vi "Auton_S3_Left_Scale.vi"   [LabVIEW 2017]
uses:
  <vilib>/Rock Robotics/WPI/Utilities/WPI_GetSetVariantRefNum.vi
  Robot Global Data.vi
  <vilib>/Rock Robotics/WPI/RobotDrive/WPI_RobotDriveArcadeDrive_Standard(NoSaturation).vi
types:
  T1 = typedef "WPI_RobotDriveDevRef.ctl" = cluster{"DevStatus":errorcluster, "Motors[]":T2[], "Square Inputs":bool, "Max Output":dbl}
  T2 = typedef "WPI_MotorControlDeviceRef.ctl" = cluster{"DeviceStatus":errorcluster, "Type":T3, "PWM":cluster{"PWM Channel":T4, "DeadBand":T5}, "CAN":cluster{"Device Number":u8, "SetOutput VI Ref":variant, "GetOutput VI Ref":variant, "Enable VI Ref":variant, "Disable VI Ref":variant, "Data":variant}, "Invert":bool, "DIO PWM":cluster{"PWM \"Enable\" Channel":T4, "DIOChannel":T6, "PWM Rate":dbl}}
  T3 = typedef "WPI_MotorControlType.ctl" = enum16{"PWM", "CAN", "DIO PWM"}
  T4 = typedef "FPGA_DIOPWMChannel.ctl" = enum8{"PWM 0", "PWM 1", "PWM 2", "PWM 3", "PWM 4", "PWM 5", "PWM 6", "PWM 7", "PWM 8", "PWM 9", "PWM MXP 0", "PWM MXP 1", "PWM MXP 2", "PWM MXP 3", "PWM MXP 4", "PWM MXP 5", "PWM MXP 6", "PWM MXP 7", "PWM MXP 8", "PWM MXP 9", "Invalid"}
  T5 = typedef "WPI_PWMDeadband.ctl" = cluster{"Name":string, "maxPositivePwm":i32, "minPositivePwm":i32, "centerPwm":i32, "maxNegativePwm":i32, "minNegativePwm":i32, "angularRange":u16}
  T6 = typedef "FPGA_DIOChannel.ctl" = enum8{"DIO 0", "DIO 1", "DIO 2", "DIO 3", "DIO 4", "DIO 5", "DIO 6", "DIO 7", "DIO 8", "DIO 9", "DIO MXP 0", "DIO MXP 1", "DIO MXP 2", "DIO MXP 3", "DIO MXP 4", "DIO MXP 5", "DIO MXP 6", "DIO MXP 7", "DIO MXP 8", "DIO MXP 9", "DIO MXP 10", "DIO MXP 11", "DIO MXP 12", "DIO MXP 13", "DIO MXP 14", "DIO MXP 15", "SPI Port CS1", "SPI Port CS2", "SPI Port CS3", "SPI Port MISO", "SPI Port MOSI", "Invalid"}
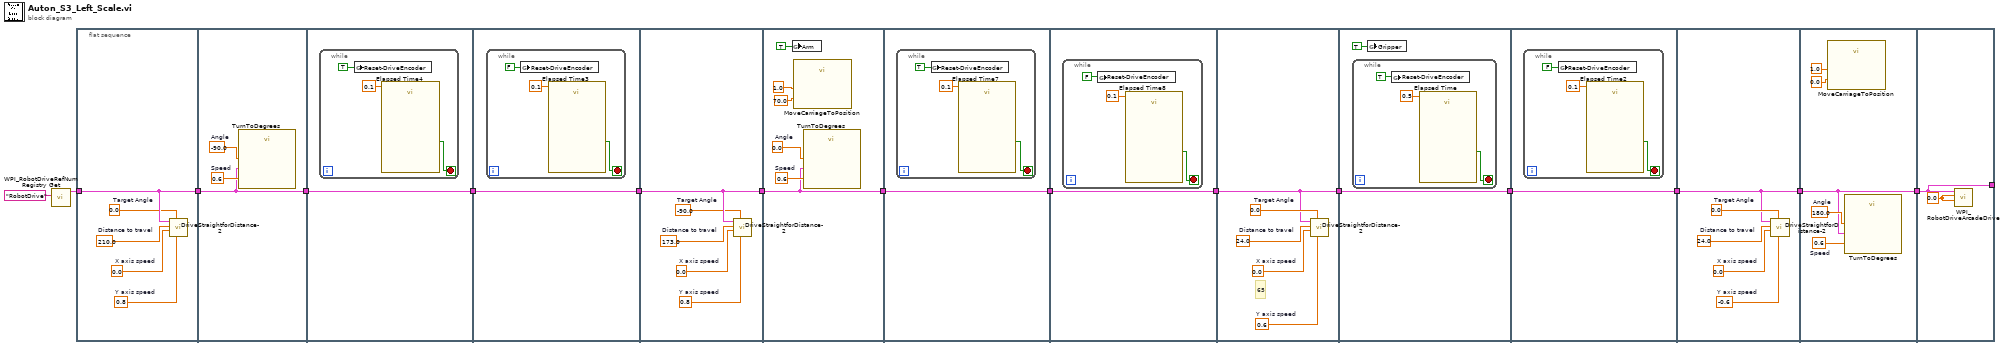
[diagram p0: block diagram]
diagram:
  n1 = call <vilib>:"WPI_RobotDriveRefNum Registry Get.vi"("refnum name"="RobotDrive") -> ("RobotDriveDevRef"=w14:T1)  [unwired: 9 in, 1 out]
  n2 = flat-sequence {
    tunnel: [w20] -> w11
    tunnel: w14 -> [w20]
    tunnel: w11 -> [w22]
    tunnel: [w22] -> w10
    tunnel: w10 -> [w24]
    tunnel: [w24] -> w12
    tunnel: w12 -> [w28]
    tunnel: [w28] -> w13
    tunnel: [w36] -> w9
    tunnel: w13 -> [w36]
    tunnel: w9 -> [w40]
    tunnel: [w40] -> w8
    tunnel: w8 -> [w43]
    tunnel: [w43] -> w7
    tunnel: w7 -> [w47]
    tunnel: [w47] -> w6
    tunnel: w6 -> [w51]
    tunnel: [w51] -> w5
    tunnel: w5 -> [w57]
    tunnel: [w57] -> w4
    tunnel: w4 -> [w61]
    tunnel: [w61] -> w3
    tunnel: w3 -> [w65]
    tunnel: [w65] -> w2
    tunnel: w2 -> [w70]
    tunnel: [w70] -> w1
    tunnel: [w75] -> _
    tunnel: w1 -> [w75]
    frame #0 {
      w16 = 0.0  # Target Angle
      w17 = 0.8  # Y axis speed
      w18 = 0.0  # X axis speed
      w19 = 210.0  # Distance to travel
      n3 = call "DriveStraightforDistance-2.vi"("Y axis speed"=w17, "Target Angle"=w16, "X axis speed"=w18, "Distance to travel"=w19, "RobotDriveDevRef"=w20) -> ()  [unwired: 7 in]
    }
    frame #1 {
      w21 = -90.0  # Angle
      w23 = 0.6  # Speed
      n4 = call "TurnToDegrees.vi"("Speed"=w23, "RobotDriveDevRef"=w22, "Angle"=w21) -> ()  [unwired: 9 in]
    }
    frame #2 {
      n5 = while {
        stop <- w27 stop-if-true
        n6 = global write "Robot Global Data.vi" "Reset-DriveEncoder"(TRUE ("Reset-DriveEncoder")) -> ()
        n7 = call "Elapsed Time4"("Time Target (s)"=0.1) -> ("Time has Elapsed"=w27:bool)  [unwired: 11 in, 7 out]
      }
    }
    frame #3 {
      n8 = while {
        stop <- w31 stop-if-true
        n9 = global write "Robot Global Data.vi" "Reset-DriveEncoder"(FALSE ("Reset-DriveEncoder")) -> ()
        n10 = call "Elapsed Time3"("Time Target (s)"=0.1) -> ("Time has Elapsed"=w31:bool)  [unwired: 11 in, 7 out]
      }
    }
    frame #4 {
      w32 = -90.0  # Target Angle
      w33 = 0.8  # Y axis speed
      w34 = 0.0  # X axis speed
      w35 = 173.0  # Distance to travel
      n11 = call "DriveStraightforDistance-2.vi"("Y axis speed"=w33, "Target Angle"=w32, "X axis speed"=w34, "Distance to travel"=w35, "RobotDriveDevRef"=w36) -> ()  [unwired: 7 in]
    }
    frame #5 {
      w41 = 0.0  # Angle
      w42 = 0.6  # Speed
      n12 = global write "Robot Global Data.vi" "Arm"(TRUE ("Arm")) -> ()
      n13 = call "MoveCarriageToPosition.vi"("Lift Speed"=1.0, "Target Height"=70.0) -> ()  [unwired: 10 in]
      n14 = call "TurnToDegrees.vi"("Speed"=w42, "RobotDriveDevRef"=w40, "Angle"=w41) -> ()  [unwired: 9 in]
    }
    frame #6 {
      n15 = while {
        stop <- w46 stop-if-true
        n16 = global write "Robot Global Data.vi" "Reset-DriveEncoder"(TRUE ("Reset-DriveEncoder")) -> ()
        n17 = call "Elapsed Time7"("Time Target (s)"=0.1) -> ("Time has Elapsed"=w46:bool)  [unwired: 11 in, 7 out]
      }
    }
    frame #7 {
      n18 = while {
        stop <- w50 stop-if-true
        n19 = global write "Robot Global Data.vi" "Reset-DriveEncoder"(FALSE ("Reset-DriveEncoder")) -> ()
        n20 = call "Elapsed Time8"("Time Target (s)"=0.1) -> ("Time has Elapsed"=w50:bool)  [unwired: 11 in, 7 out]
      }
    }
    frame #8 {
      w52 = 0.0  # Target Angle
      w53 = 0.6  # Y axis speed
      w54 = 0.0  # X axis speed
      w55 = 24.0  # Distance to travel
      # "65"
      n21 = call "DriveStraightforDistance-2.vi"("Y axis speed"=w53, "Target Angle"=w52, "X axis speed"=w54, "Distance to travel"=w55, "RobotDriveDevRef"=w51) -> ()  [unwired: 7 in]
    }
    frame #9 {
      n22 = while {
        stop <- w60 stop-if-true
        n23 = global write "Robot Global Data.vi" "Reset-DriveEncoder"(TRUE ("Reset-DriveEncoder")) -> ()
        n24 = call "Elapsed Time"("Time Target (s)"=0.5) -> ("Time has Elapsed"=w60:bool)  [unwired: 11 in, 7 out]
      }
      n25 = global write "Robot Global Data.vi" "Gripper"(TRUE ("Gripper")) -> ()
    }
    frame #10 {
      n26 = while {
        stop <- w64 stop-if-true
        n27 = global write "Robot Global Data.vi" "Reset-DriveEncoder"(FALSE ("Reset-DriveEncoder")) -> ()
        n28 = call "Elapsed Time2"("Time Target (s)"=0.1) -> ("Time has Elapsed"=w64:bool)  [unwired: 11 in, 7 out]
      }
    }
    frame #11 {
      w66 = 0.0  # Target Angle
      w67 = -0.6  # Y axis speed
      w68 = 0.0  # X axis speed
      w69 = 24.0  # Distance to travel
      n29 = call "DriveStraightforDistance-2.vi"("Y axis speed"=w67, "Target Angle"=w66, "X axis speed"=w68, "Distance to travel"=w69, "RobotDriveDevRef"=w65) -> ()  [unwired: 7 in]
    }
    frame #12 {
      w73 = 180.0  # Angle
      w74 = 0.6  # Speed
      n30 = call "MoveCarriageToPosition.vi"("Lift Speed"=1.0, "Target Height"=0.0) -> ()  [unwired: 10 in]
      n31 = call "TurnToDegrees.vi"("Speed"=w74, "RobotDriveDevRef"=w70, "Angle"=w73) -> ()  [unwired: 9 in]
    }
    frame #13 {
      w76 = 0.0 ("X axis value")
      n32 = call-poly <vilib>:"WPI_RobotDriveArcadeDrive.vi"("Y axis value"=w76, "X axis value"=w76, "RobotDriveDevRef"=w75) -> ()  [unwired: 6 in, 3 out]
    }
  }
